vi "NF87XX.get acceleration.vi"(0 "i ref in":refnum<vi>, 2 "System":string="N/A", 5 "error in (no error)":errorcluster) -> (14 "i ref out":refnum<vi>, 16 "acceleration Mot 0 [steps/s²]":dbl, 17 "acceleration Mot 1 [steps/s²]":dbl, 18 "acceleration Mot 2 [steps/s²]":dbl, 19 "error out":errorcluster)   [LabVIEW 2014, in "NF87XX.lvlib"]
doc: "Gets the acceleration from all systems (drivers) and writes it to own attributes. Returns the acceleration of up to 3 motors in Steps/s² if \"System\" is found to be one of the driver names. Thereby 99999 indicates that an error occured or the value is not available.\n\nauthor: Stefan Götte\ndata: 09-JAN-2007\n\n\n\n\nLicense Agreement for this software:\n\nCopyright (C)\nGesellschaft für Schwerionenforschung, GSI\nPlanckstr. 1\n64291 Darmstadt\nGermany\n\nContact: D.Beck@gsi.de \n\nThis program is free software; you can redistribute it and/or modify it under the terms of the GNU General Public License as published by the Free Software Foundation; either version 2 of the license, or (at your option) any later version.\n\nThis program is distributed in the hope that it will be useful, but WITHOUT ANY WARRANTY; without even the implied warranty of MERCHANTABILITY or FITNESS FOR A PARTICULAR PURPOSE. See the GNU General License for more details (http://www.gnu.org).\n\nGesellschaft für Schwerionenforschung, GSI\nPlanckstr. 1, 64291 Darmstadt, Germany\nFor all questions and ideas contact: M.Richter@gsi.de, H.Brand@gsi.de or D.Beck@gsi.de.\nLast update: 17-JUN-2004"
uses:
  NF87XX.lvlib
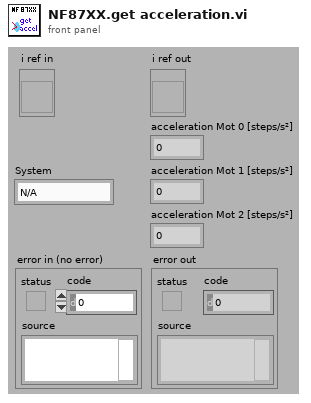
[diagram p1: front panel]
types:
  T1 = enum16{"User....", "DEF", "DIAG", "INI", "LOCK", "UNLOCK", "MAP", "SAV", "VER", "ACC", "CHL", "FOR", "GO", "HAL", "MOF", "MON", "MPV", "POS", "REL", "REV", "STA", "STO", "TYP", "VEL", "ABS", "SER", "NOS", "DRT", "FLI", "RLI", "FIN", "RIN", "AIN", "IN", "JOF", "JON", "OUT", "RES FINE", "RES COARSE", "02 (HEX)", "PWM", "CNT", "TMR", "HOSTNAME", "IPADDR", "IPMODE", "NETMASK", "GATEWAY", "DNSSRVR", "PASSWD", "ECHO", "MACADDR"}
  T2 = typedef "NF87XX.lvlib/NF87XX.i attribute.ctl" = cluster{"Con Settings":T3, "Drivers":T4[], "Status":cluster{"Service ID":i32, "Status":T7}, "Joystick available":bool, "VISA Resource":string}
  T3 = typedef "NewFocusPico - Driver np.lvlib/VISA & TCPIP Control.ctl" = cluster{"VISA or TCP/IP":bool, "Init Connection":bool, "Close Connection":bool, "Resource Name":refnum<visa-resource-name>, "hostname":string, "connection ID":refnum<k5>}
  T4 = typedef "NF87XX.lvlib/NF87XX.driver Settings.ctl" = cluster{"Name":string, "Driver Type":T5, "Pico Parameter type":T6, "Acceleration [Steps/s²]":cluster{"Motor 0":dbl, "Motor 1":dbl, "Motor 2":dbl}, "Start Velocity [Steps/s]":cluster{"Motor 0":dbl, "Motor 1":dbl, "Motor 2":dbl}, "Velocity [Steps/s]":cluster{"Motor 0":dbl, "Motor 1":dbl, "Motor 2":dbl}, "axis channel":i32, "Position":i32, "Position Service ID":i32}
  T5 = typedef "NF87XX.lvlib/NF87XX.driver Type.ctl" = enum16{"not defined", "3-ch open loop drv", "1-ch closed loop drv"}
  T6 = typedef "NewFocusPico - Driver np.lvlib/Pico Parameters.ctl" = cluster{"Pico Type":enum16{"Open-Loop Pico", "Close-Loop Pico", "Pico Ultra"}, "Acceleration (steps/sec^2)":string, "Velocity ( Hz)":string, "Driver":string, "Motor":string, "Channel":string, "Process Step":string}
  T7 = typedef "PH_StatusHandler.lvlib/PH_StatusHandler.Status.ctl" = i16
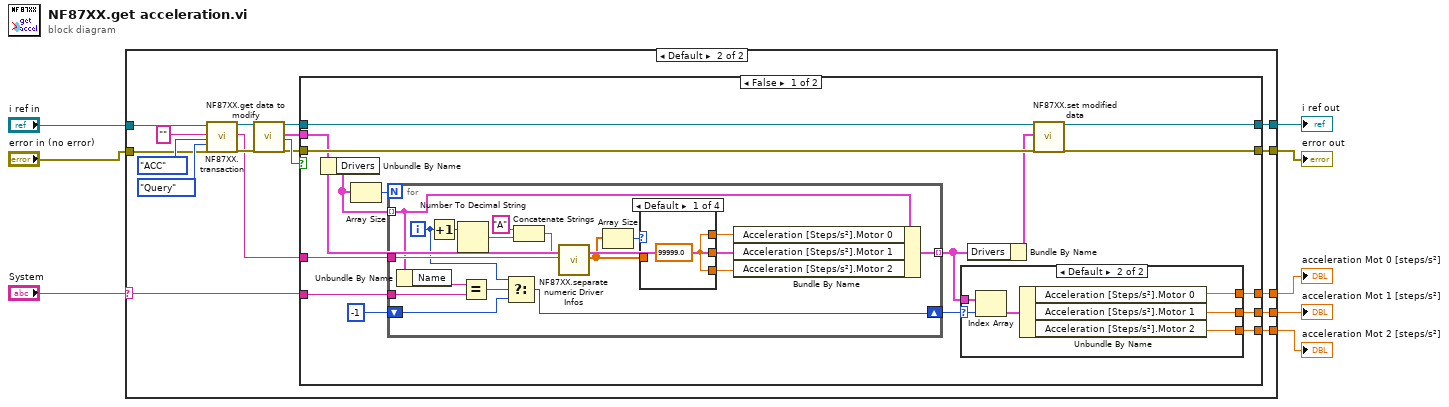
[diagram p0: block diagram]
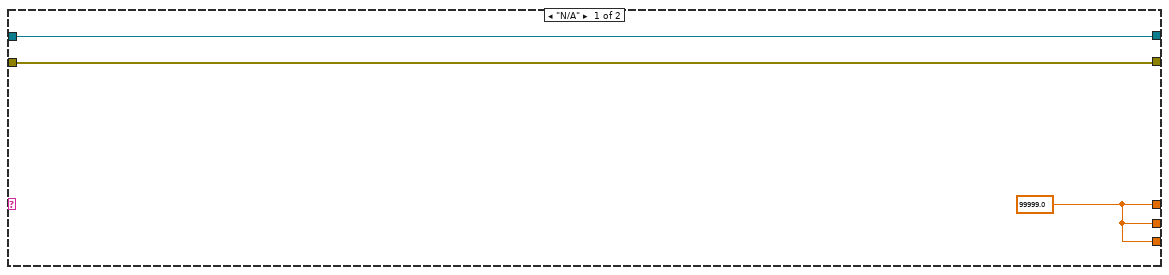
[diagram p2: hidden frame]
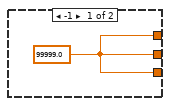
[diagram p3: hidden frame]
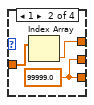
[diagram p4: hidden frame]
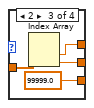
[diagram p5: hidden frame]
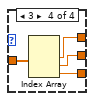
[diagram p6: hidden frame]
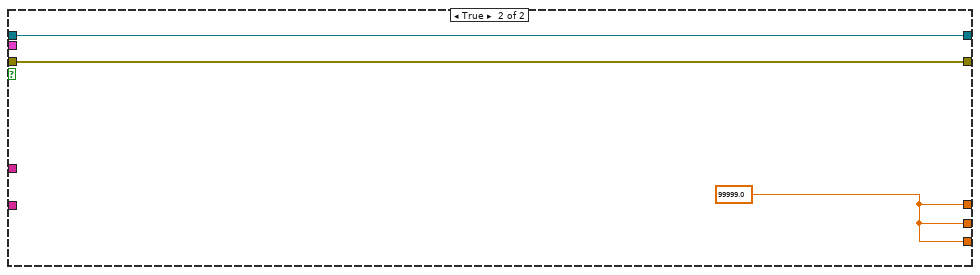
[diagram p7: hidden frame]
diagram:
  n1 = case shown="Default" "System" {
    selector: "System" -> [_ w12]
    tunnel: "i ref in" -> [w11 w26]
    tunnel: "error in (no error)" -> [w10 w25]
    tunnel: [w11 w17] -> w6
    tunnel: [w10 w16] -> w5
    tunnel: [w9 w15] -> w4
    tunnel: [w9 w14] -> w3
    tunnel: [w9 w13] -> w2
    frame "N/A" {
      w9 = 99999.0 ("Motor 0")
    }
    frame Default {
      n2 = call "NF87XX.transaction.vi"("i ref in"=w26, "User Cmd/Numeric Argu"="", "MCL Cmd"=T1."ACC", "Query/Set"=enum16{"Query", "Set"}."Query", "error in (no error)"=w25) -> ("i ref out"=w19:refnum<vi>, "Read String"=w18:string, "error out"=w20:errorcluster)  [unwired: 12 in]
      n3 = call "NF87XX.get data to modify.vi"("i ref in"=w19, "error in (no error)"=w20) -> ("i ref out"=w23:refnum<vi>, "i attribute"=w22:T2, "timed out"=w24:bool, "error out"=w21:errorcluster)  [unwired: 14 in]
      n4 = case shown="False" w24 {
        tunnel: w23 -> [w45 w85]
        tunnel: w22 -> [w39 _]
        tunnel: [w42 w85] -> w17
        tunnel: w21 -> [w44 w84]
        tunnel: [w43 w84] -> w16
        tunnel: w18 -> [w41 _]
        tunnel: w12 -> [w36 _]
        tunnel: [w33 w83] -> w14
        tunnel: [w32 w83] -> w15
        tunnel: [w31 w83] -> w13
        frame False {
          n5 = Unbundle By Name(w39) -> ("Drivers"=w35:T4[])
          n6 = Array Size(array=w35) -> (size(s)=w40:i32)
          n7 = for {
            N: w40 -> [_]
            tunnel: w41 -> [w70]
            tunnel: w35 -> [w54] mode=indexing
            tunnel: [w53] -> w37 mode=indexing
            tunnel: w36 -> [w61]
            shift-right: [w62] -> w30
            shift-left: -1 -> [w58]
            i -> [w59]
            n8 = Unbundle By Name(w54) -> ("Name"=w60:string)
            n9 = Increment(x=w59) -> (x+1=w69:i32)
            n10 = Number To Decimal String(number=w69) -> (decimal integer string=w67:string)  [unwired: 1 in]
            n11 = Equal?(x=w60, y=w61) -> (x = y?=w63:bool)
            n12 = Select(t=w59, s=w63, f=w58) -> (s? t:f=w62:i32)
            n13 = Concatenate Strings("A" ("string"), w67) -> (w66:string)
            n14 = call "NF87XX.separate numeric Driver Infos.vi"("Driver"=w66, "Read String"=w70) -> ("Result"=w64:dbl[])  [unwired: 17 in]
            n15 = Array Size(array=w64) -> (size(s)=w65:i32)
            n16 = case shown="Default" w65 {
              tunnel: w64 -> [_ w74 w78 w82]
              tunnel: [w71 w73 w77 w81] -> w57
              tunnel: [w71 w72 w76 w80] -> w56
              tunnel: [w71 w72 99999.0 w79] -> w55
              frame Default {
                w71 = 99999.0
              }
              frame 1 {
                w72 = 99999.0
                n17 = Index Array(array=w74) -> (element=w73:dbl)  [unwired: 1 in]
              }
              frame 2 {
                n18 = Index Array(array=w78) -> (element #1=w77:dbl, element #2=w76:dbl)  [unwired: 2 in]
              }
              frame 3 {
                n19 = Index Array(array=w82) -> (element #1=w81:dbl, element #2=w80:dbl, element #3=w79:dbl)  [unwired: 3 in]
              }
            }
            n20 = Bundle By Name(cluster=w54, "Acceleration [Steps/s²].Motor 0"=w57, "Acceleration [Steps/s²].Motor 1"=w56, "Acceleration [Steps/s²].Motor 2"=w55) -> (w53:T4)
          }
          n21 = case shown="Default" w30 {
            selector: w30 -> [_ w47]
            tunnel: w37 -> [_ w52]
            tunnel: [w46 w50] -> w33
            tunnel: [w46 w49] -> w32
            tunnel: [w46 w48] -> w31
            frame -1 {
              w46 = 99999.0 ("Motor 1")
            }
            frame Default {
              n22 = Index Array(array=w52, index=w47) -> (element=w51:T4)
              n23 = Unbundle By Name(w51) -> ("Acceleration [Steps/s²].Motor 0"=w50:dbl, "Acceleration [Steps/s²].Motor 1"=w49:dbl, "Acceleration [Steps/s²].Motor 2"=w48:dbl)
            }
          }
          n24 = Bundle By Name(cluster=w39, "Drivers"=w37) -> (w38:T2)
          n25 = call "NF87XX.set modified data.vi"("i ref in"=w45, "i attribute"=w38, "error in (no error)"=w44) -> ("i ref out"=w42:refnum<vi>, "error out"=w43:errorcluster)  [unwired: 15 in]
        }
        frame True {
          w83 = 99999.0 ("Motor 0")
        }
      }
    }
  }
  "error out" <- w5
  "i ref out" <- w6
  "acceleration Mot 0 [steps/s²]" <- w3
  "acceleration Mot 1 [steps/s²]" <- w4
  "acceleration Mot 2 [steps/s²]" <- w2
